vi "串口关闭.vi"(1 "错误输入（无错误）":errorcluster, 2 "VISA资源名称":refnum<visa-resource-name>) -> ()   [LabVIEW 2019]
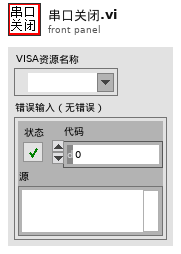
[diagram p1: front panel]
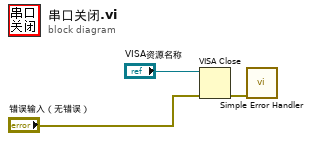
[diagram p0: block diagram]
diagram:
  n1 = VISA Close(VISA resource name="VISA资源名称", error in (no error)="错误输入（无错误）") -> (error out=w3:errorcluster)
  n2 = call <vilib>:"Simple Error Handler.vi"("error in (no error)"=w3) -> ()  [unwired: 1 in, 8 out]
